vi "Set Reentrancy for Selected VIs.vi"(6 "Reentrancy Type":T1(ring), 8 "error in":errorcluster, 9 "Is Reentrant":bool, 10 "Selected VIs":string[](array[string]), 11 "Application in":refnum<vi>) -> (0 "error out":errorcluster)   [LabVIEW 2013, in "LVTM.lvlib"]
uses:
  LVTM.lvlib
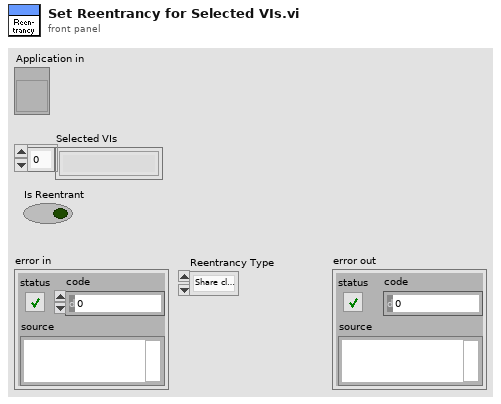
[diagram p1: front panel]
types:
  T1 = enum16{"Share clones between instances", "Preallocate clone for each instance"}
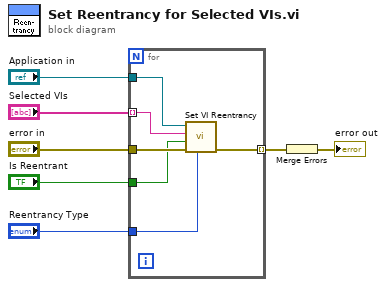
[diagram p0: block diagram]
diagram:
  n1 = for {
    tunnel: [w13] -> w3 mode=indexing
    tunnel: "error in" -> [w11]
    tunnel: "Selected VIs" -> [w10] mode=indexing
    tunnel: "Application in" -> [w12]
    tunnel: "Reentrancy Type" -> [w9]
    tunnel: "Is Reentrant" -> [w8]
    n2 = call "Set VI Reentrancy.vi"("Reentrancy Type"=w9, "error in (no error)"=w11, "Is Reentrant"=w8, "VI Name"=w10, "Application Reference"=w12) -> ("error out"=w13:errorcluster)  [unwired: 6 in]
  }
  n3 = Merge Errors(w3) -> (→"error out":errorcluster)
